vi "WDT FIFO Waveforms DBL.vi"(7 "FIFO":i32, 8 "error in (no error)":errorcluster, 9 "Hammer":waveform(dbl), 10 "Triggered?":bool, 11 "Mic":waveform(dbl)) -> (0 "error out":errorcluster, 1 "Hammer out":waveform(dbl), 2 "Full":bool, 3 "Mic out":waveform(dbl))   [LabVIEW 2022 SP3]
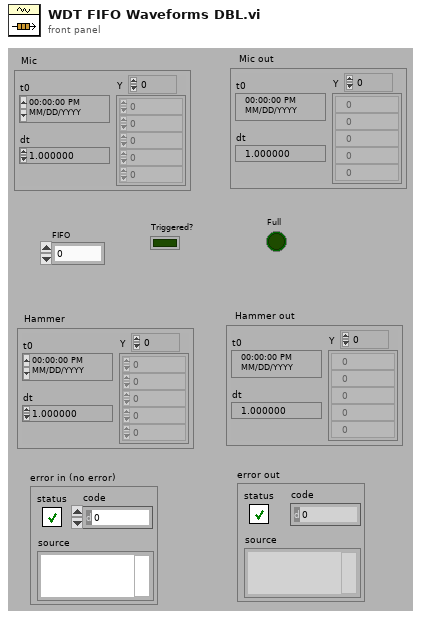
[diagram p1: front panel]
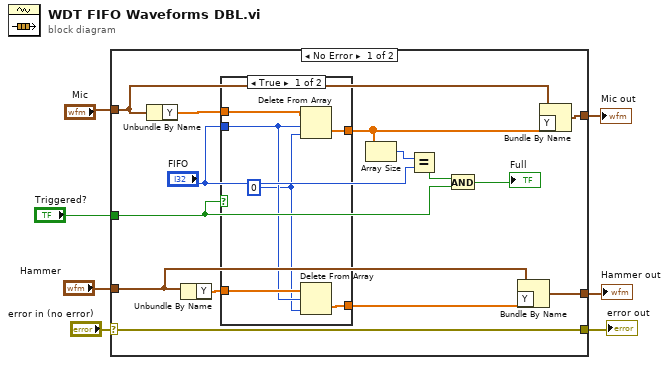
[diagram p0: block diagram]
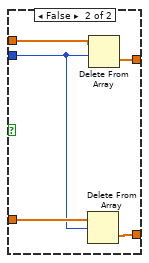
[diagram p2: hidden frame]
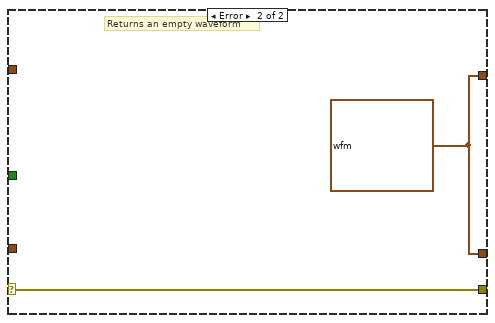
[diagram p3: hidden frame]
diagram:
  n1 = case shown="No Error" "error in (no error)" {
    selector: "error in (no error)" -> [w19 w34]
    tunnel: "Mic" -> [w21 _]
    tunnel: [w20 w33] -> w7
    tunnel: [w19 w34] -> w4
    tunnel: "Hammer" -> [w18 _]
    tunnel: [w17 w33] -> w2
    tunnel: "Triggered?" -> [w8 _]
    frame No Error {
      n2 = Unbundle By Name(w21) -> ("Y"=w16:dbl[])
      n3 = Unbundle By Name(w18) -> ("Y"=w13:dbl[])
      n4 = case shown="True" w8 {
        tunnel: w16 -> [w27 w32]
        tunnel: [w26 w31] -> w15
        tunnel: w13 -> [w25 w30]
        tunnel: "FIFO" -> [w23 w28]
        tunnel: [w24 w29] -> w11
        frame True {
          w22 = 0 ("index")
          n5 = Delete From Array(array=w27, length=w23, index=w22) -> (deleted portion=w26:dbl[])  [unwired: 1 out]
          n6 = Delete From Array(array=w25, length=w23, index=w22) -> (deleted portion=w24:dbl[])  [unwired: 1 out]
        }
        frame False {
          n7 = Delete From Array(array=w30, length=w28) -> (deleted portion=w29:dbl[])  [unwired: 1 in, 1 out]
          n8 = Delete From Array(array=w32, length=w28) -> (deleted portion=w31:dbl[])  [unwired: 1 in, 1 out]
        }
      }
      n9 = Array Size(array=w15) -> (size(s)=w14:i32)
      n10 = Equal?(x=w14, y="FIFO") -> (x = y?=w10:bool)
      n11 = And(x=w10, y=w8) -> (x .and. y?=→"Full":bool)
      n12 = Bundle By Name(cluster=w18, "Y"=w11) -> (w17:waveform(dbl))
      n13 = Bundle By Name(cluster=w21, "Y"=w15) -> (w20:waveform(dbl))
    }
    frame Error {
      w33 = waveform(dbl) {"t0"=timestamp(0 s since 1904-01-01), "dt"=0.0, "Y"=[]} ("waveform B")
      # "Returns an empty waveform"
      # "Incoming Error"
    }
  }
  "Mic out" <- w7
  "error out" <- w4
  "Hammer out" <- w2
